vi "Query Local Node Identity.vi"(8 "error in (no error)":errorcluster, 11 "VISA resource name":refnum<visa-resource-name>) -> (0 "error out":errorcluster, 1 "Serial Number":string, 2 "Model":string, 3 "VISA resource name out":refnum<visa-resource-name>, 5 "Firmware Revision":string)   [LabVIEW 2019, in "Keithley 2600 Series.lvlib"]
doc: "Returns the instrument's model number, firmware revision and serial number."
uses:
  Keithley 2600 Series.lvlib
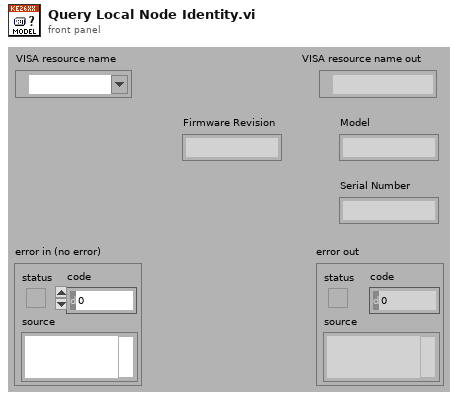
[diagram p1: front panel]
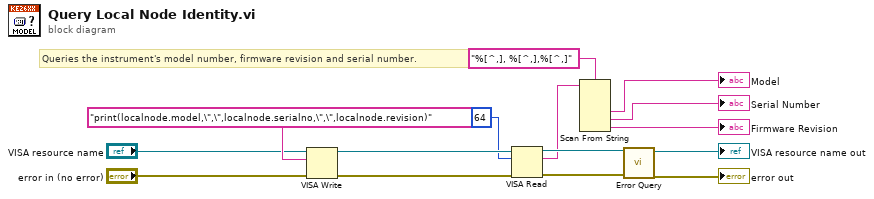
[diagram p0: block diagram]
diagram:
  # "Queries the instrument's model number, firmware revision and serial number."
  n1 = VISA Write(VISA resource name="VISA resource name", write buffer="print(localnode.model,\",\",localnode.serialno,\",\",localnode.revision)", error in (no error)="error in (no error)") -> (VISA resource name out=w10:refnum<visa-resource-name>, error out=w9:errorcluster)  [unwired: 1 out]
  n2 = VISA Read(VISA resource name=w10, byte count=u32 64, error in (no error)=w9) -> (VISA resource name out=w8:refnum<visa-resource-name>, read buffer=w5:string, error out=w7:errorcluster)  [unwired: 1 out]
  n3 = Scan From String(format string="%[^,], %[^,],%[^,]", input string=w5) -> (output 1=→"Model":string, output 2=→"Serial Number":string, output 3=→"Firmware Revision":string)  [unwired: 5 in, 3 out]
  n4 = call "Error Query.vi"("error in (no error)"=w7, "VISA resource name"=w8) -> ("error out"=→"error out":errorcluster, "VISA resource name out"=→"VISA resource name out":refnum<visa-resource-name>)  [unwired: 6 in, 2 out]
